vi "GetControlModuleVersion.vi"(8 "error in":errorcluster, 10 "control module number":T1=1 items=["control module 1"=1, "control module 2"=2, "control module 3"=3, "control module 4"=4], 11 "VISA resource name":refnum<visa-resource-name>) -> (0 "error out":errorcluster, 2 "version number of control module":string, 3 "VISA resource name out":refnum<visa-resource-name>)   [LabVIEW 2023, in "Thermotron 8800.lvlib"]
doc: "CMVR\nCommand name: Send version number of control module\nCommand type: System status\nDescription: This command retrieves the version number of the specified control module.\nQuery syntax: CMVRcm?\nWhere cm = control module (1 through 4)\nQuery example: CMVR2?\n8800 response: V2.18 09/06/11 (Control module 2 is version 2.18, released September 6, 2011.)"
uses:
  Thermotron 8800.lvlib
  Private/control module number.ctl
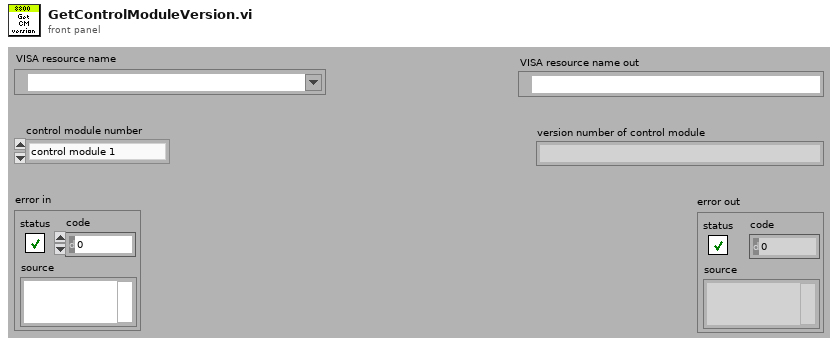
[diagram p1: front panel]
types:
  T1 = typedef "Thermotron 8800.lvlib/control module number.ctl" = u16
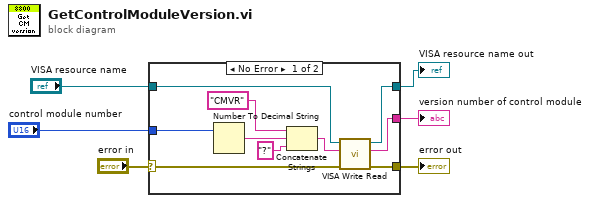
[diagram p0: block diagram]
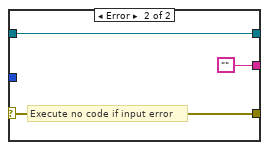
[diagram p2: hidden frame]
diagram:
  n1 = case shown="No Error" "error in" {
    selector: "error in" -> [w11 w18]
    tunnel: "control module number" -> [w12 _]
    tunnel: [w10 w18] -> w4
    tunnel: "VISA resource name" -> [w9 w19]
    tunnel: [w8 w19] -> w2
    tunnel: [w7 ""] -> w1
    frame No Error {
      n2 = Number To Decimal String(number=w12) -> (decimal integer string=w13:string)  [unwired: 1 in]
      n3 = Concatenate Strings("CMVR" ("8800 Command"), w13, "?" ("8800 Command")) -> (w16:string)
      n4 = call "VISA Write Read.vi"("error in (no error)"=w11, "8800 Command"=w16, "VISA Refnum in"=w9) -> ("error out"=w10:errorcluster, "read buffer"=w7:string, "VISA Refnum out"=w8:refnum<visa-resource-name>)  [unwired: 6 in]
    }
    frame Error {
      # "Execute no code if input error"
    }
  }
  "error out" <- w4
  "VISA resource name out" <- w2
  "version number of control module" <- w1
